vi "Substitute Class.vi"(8 "error in (no error)":errorcluster, 10 "New Class":path=path "C:/temp/Test2/Test2.lvclass", 11 "Class to Replace":path=path "C:/temp/Test1.lvclass") -> (0 "error out":errorcluster)   [LabVIEW 2020, in "Mock Class Updater.lvclass"]
uses:
  Mock Class Updater.lvclass
  Mock Class Updater.lvclass/Mock Class Updater.ctl
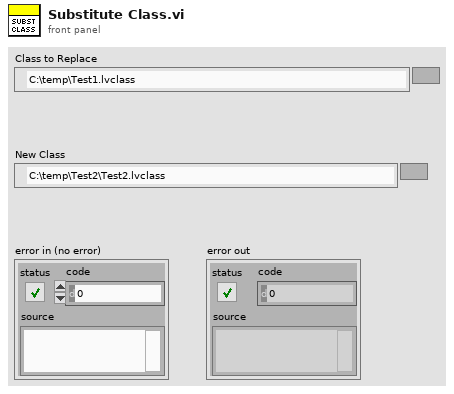
[diagram p1: front panel]
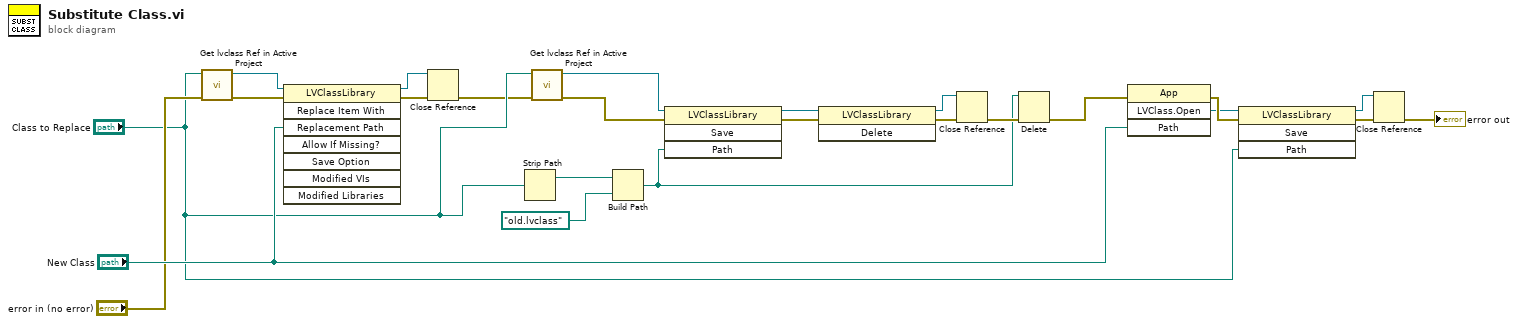
[diagram p0: block diagram]
diagram:
  n1 = call "Get lvclass Ref in Active Project.vi"("error in (no error)"="error in (no error)", "Class to Replace"="Class to Replace") -> ("error out"=w17:errorcluster, "LVClassLibrary out"=w18:refnum<vi>)  [unwired: 8 in]
  n2 = invoke class="LVClassLibrary" method="Replace Item With"(reference=w18, error in=w17, "Replacement Path"="New Class") -> (reference out=w11:refnum<vi>, error out=w15:errorcluster)  [unwired: 5 in, 6 out]
  n3 = Close Reference(reference=w11, error in (no error)=w15) -> (error out=w7:errorcluster)
  n4 = Strip Path(path="Class to Replace") -> (stripped path=w13:path)  [unwired: 1 out]
  n5 = call "Get lvclass Ref in Active Project.vi"("error in (no error)"=w7, "Class to Replace"="Class to Replace") -> ("error out"=w6:errorcluster, "LVClassLibrary out"=w5:refnum<vi>)  [unwired: 8 in]
  n6 = Build Path(base path=w13, name or relative path=path "old.lvclass") -> (appended path=w1:path)
  n7 = invoke class="LVClassLibrary" method="Save"(reference=w5, error in=w6, "Path"=w1) -> (reference out=w9:refnum<vi>, error out=w14:errorcluster)  [unwired: 1 in, 2 out]
  n8 = invoke class="LVClassLibrary" method="Delete"(reference=w9, error in=w14) -> (reference out=w3:refnum<vi>, error out=w10:errorcluster)  [unwired: 1 in, 1 out]
  n9 = Close Reference(reference=w3, error in (no error)=w10) -> (error out=w4:errorcluster)
  n10 = Delete(path (use dialog)=w1, error in=w4) -> (error out=w2:errorcluster)  [unwired: 3 in, 2 out]
  n11 = invoke class="App" method="LVClass.Open"(error in=w2, "Path"="New Class") -> (error out=w20:errorcluster, "LVClass.Open"=w19:refnum<vi>)  [unwired: 2 in, 2 out]
  n12 = invoke class="LVClassLibrary" method="Save"(reference=w19, error in=w20, "Path"="Class to Replace") -> (reference out=w23:refnum<vi>, error out=w21:errorcluster)  [unwired: 1 in, 2 out]
  n13 = Close Reference(reference=w23, error in (no error)=w21) -> (error out=→"error out":errorcluster)
